vi "DataReadBinGen.vi"(0 "error in":errorcluster, 2 "Index (0)":i64, 3 "chemin Data":path) -> (5 "DernColVal":i32, 6 "error out":errorcluster, 7 "LastScanPos":dbl[](array[numeric]), 8 "XY Graph":T1(array[cluster]), 9 "AllYData":dbl[][](array[numeric]) format="%#.3f")   [LabVIEW 2010]
doc: "Ce VI lit les données contenu dans le fichier de sauvegarde automatique. Ces données correspondent aux valeurs prises lors du dernier balayage. La sauvegarde automatique est effectué après chaque acquisition."
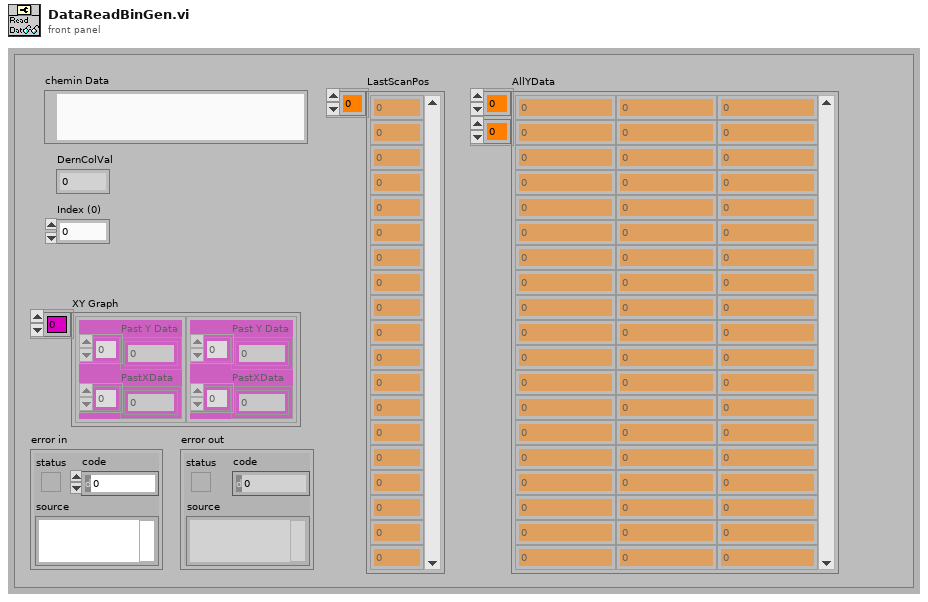
[diagram p1: front panel]
types:
  T1 = cluster{"Past Y Data":dbl[], "PastXData":dbl[]}[]
  T2 = cluster{"AllYData 2":dbl[][], "XY Graph":cluster{"Past Y Data":dbl[], "PastXData":dbl[]}[], "LastScanPos 2":dbl[]}
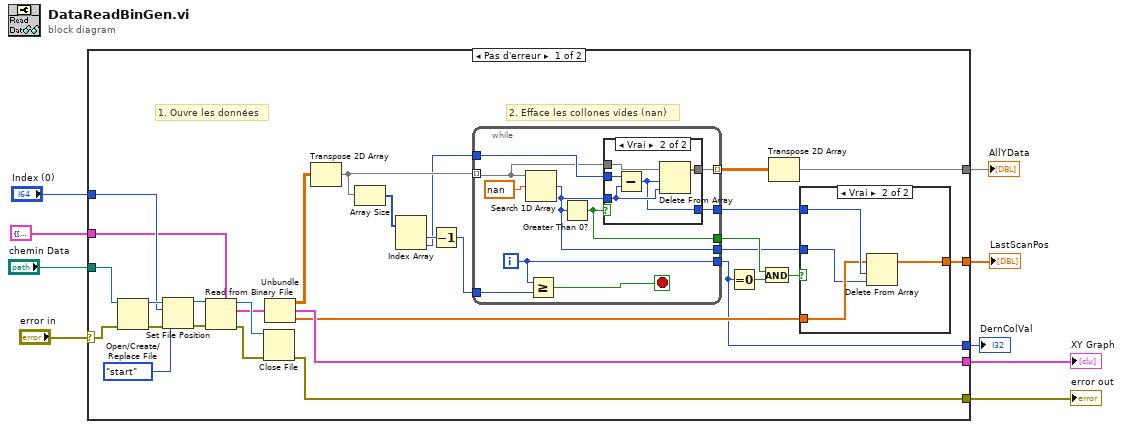
[diagram p0: block diagram]
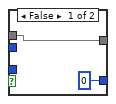
[diagram p3: hidden frame]
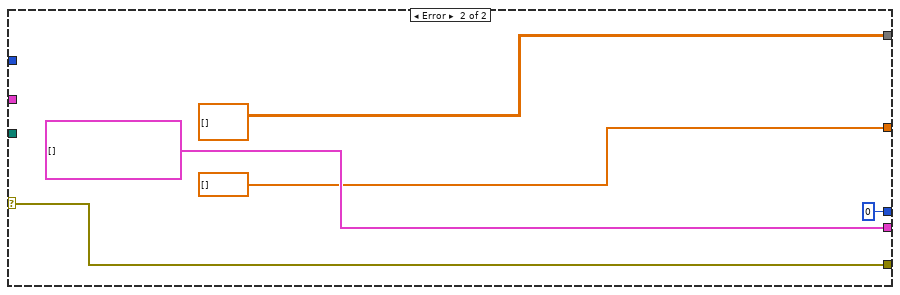
[diagram p4: hidden frame]
diagram:
  n1 = case shown="Pas d'erreur" "error in" {
    selector: "error in" -> [w36 w63]
    tunnel: "chemin Data" -> [w39 _]
    tunnel: T2 {"AllYData 2"=[], "XY Graph"=[], "LastScanPos 2"=[]} ("output cluster") -> [w10 _]
    tunnel: [w35 w63] -> w8
    tunnel: [w24 dbl[][] [] ("AllYData 2")] -> w7
    tunnel: [w37 T1 [] ("XY Graph")] -> w4
    tunnel: [w27 dbl[] [] ("LastScanPos 2")] -> w6
    tunnel: [w19 0] -> w3
    tunnel: "Index (0)" -> [w13 _]
    frame No Error {
      # "2. Efface les collones vides (nan)"
      # "1. Ouvre les données"
      n2 = Open/Create/Replace File(file path (use dialog)=w39, error in=w36) -> (refnum out=w16:refnum<file>, error out=w15:errorcluster)  [unwired: 4 in, 1 out]
      n3 = Set File Position(offset (in bytes) (0)=w13, refnum=w16, from (0:start)=enum16{"start", "end", "current"}."start" ("à partir de (0 : start)"), error in=w15) -> (refnum out=w17:refnum<file>, error out=w14:errorcluster)
      n4 = Read from Binary File(5:w10, 8:w14, 11:w17) -> (0:w38:errorcluster, 2:w11:T2, 3:w34:refnum<file>)  [unwired: 3 in, 1 out]
      n5 = Close File(refnum=w34, error in=w38) -> (error out=w35:errorcluster)  [unwired: 1 out]
      n6 = Unbundle(w11) -> ("AllYData 2"=w28:dbl[][], "XY Graph"=w37:T1, "LastScanPos 2"=w29:dbl[])
      n7 = Transpose 2D Array(2D array=w28) -> (transposed array=w30:dbl[][])
      n8 = Array Size(array=w30) -> (size(s)=w33:i32[])
      n9 = Index Array(array=w33) -> (element #1=w32:i32, element #2=w26:i32)  [unwired: 2 in]
      n10 = Decrement(x=w32) -> (x-1=w31:i32)
      n11 = while {
        tunnel: w30 -> [w50] mode=indexing
        tunnel: [w52] -> w19
        tunnel: w31 -> [w53]
        tunnel: w26 -> [w51]
        tunnel: [w49] -> w25 mode=indexing
        tunnel: [w48] -> w18
        tunnel: [w46] -> w22
        tunnel: [w47] -> w20
        i -> [w52]
        stop <- w45 stop-if-true
        n12 = Search 1D Array(1D array=w50, element=nan ("élément")) -> (index of element=w48:i32)  [unwired: 1 in]
        n13 = Greater Or Equal?(x=w52, y=w53) -> (x >= y?=w45:bool)
        n14 = Greater Than 0?(x=w48) -> (x > 0?=w46:bool)
        n15 = case shown="Vrai" w46 {
          tunnel: w51 -> [_ w61]
          tunnel: w48 -> [_ w59]
          tunnel: w50 -> [w56 w60]
          tunnel: [w56 w58] -> w49
          tunnel: [0 w57] -> w47
          frame False {
          }
          frame True {
            n16 = Subtract(x=w61, y=w59) -> (x-y=w57:i32)
            n17 = Delete From Array(array=w60, length=w57, index=w59) -> (array with subset deleted=w58:dbl[])  [unwired: 1 out]
          }
        }
      }
      n18 = Equal To 0?(x=w19) -> (x = 0?=w23:bool)
      n19 = And(x=w22, y=w23) -> (x .and. y?=w21:bool)
      n20 = Transpose 2D Array(2D array=w25) -> (transposed array=w24:dbl[][])
      n21 = case shown="Vrai" w21 {
        tunnel: w29 -> [w40 w43]
        tunnel: [w40 w42] -> w27
        tunnel: w20 -> [_ w44]
        tunnel: w18 -> [_ w41]
        frame False {
        }
        frame True {
          n22 = Delete From Array(array=w43, length=w44, index=w41) -> (array with subset deleted=w42:dbl[])  [unwired: 1 out]
        }
      }
    }
    frame Error {
    }
  }
  "error out" <- w8
  "AllYData" <- w7
  "LastScanPos" <- w6
  "XY Graph" <- w4
  "DernColVal" <- w3
